vi "Analog IO.vi"(4 "R Audio In":i16, 5 "C O/P":i16[](array[numeric])=[0, 0], 6 "B O/P":u16[](array[numeric])=[0, 0, 0, 0], 7 "A O/P":u16[](array[numeric])=[0, 0, 0, 0]) -> (0 "R Audio Out":i16, 1 "C I/P":i16[](array[numeric]), 2 "B I/P":i16[](array[numeric]), 3 "A I/P":u16[](array[numeric]))   [LabVIEW 2015]
uses:
  <vilib>/rvi/eio/common/nirviEmuTemplateMethod_errors.vi
  <vilib>/eio/EIONode/EIONode.xnode
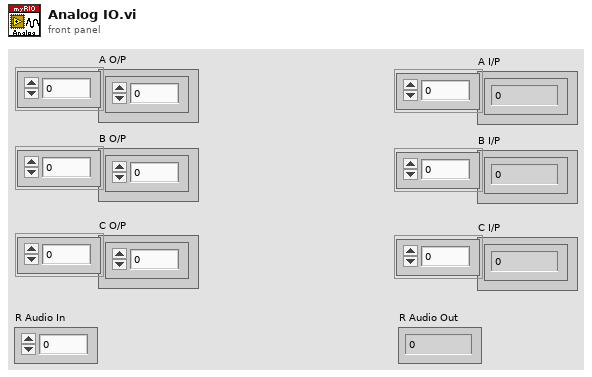
[diagram p1: front panel]
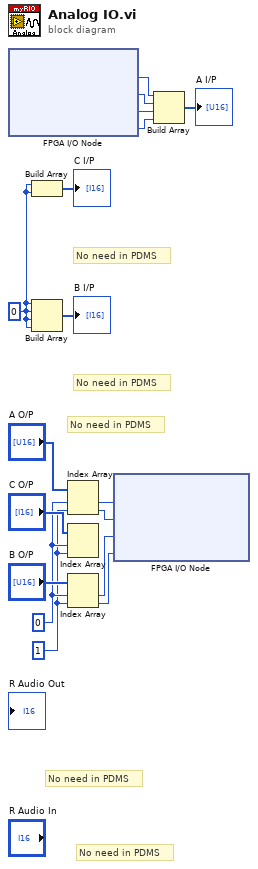
[diagram p0: block diagram]
diagram:
  w1 = i16 0
  w6 = i16 1
  w7 = i16 0
  # "No need in PDMS"
  # "No need in PDMS"
  # "No need in PDMS"
  # "No need in PDMS"
  # "No need in PDMS"
  n1 = xnode "FPGA I/O Node"() -> ("ConnectorA/AI0"=w17:u16, "ConnectorA/AI1"=w13:u16, "ConnectorA/AI2"=w12:u16, "ConnectorA/AI3"=w11:u16)  [unwired: 4 in, 4 out]
  n2 = Build Array(w1, w1) -> (→"C I/P":i16[])
  n3 = Build Array(w1, w1, w1, w1) -> (→"B I/P":i16[])
  n4 = Index Array(array="A O/P", index #1=w7, index #2=w6) -> (element #1=w5:u16, element #2=w4:u16)
  n5 = Index Array(array="C O/P", index #1=w7, index #2=w6) -> ()  [unwired: 2 out]
  n6 = Index Array(array="B O/P", index #1=w7, index #2=w6) -> (element #1=w3:u16, element #2=w2:u16)
  n7 = xnode "FPGA I/O Node"("ConnectorA/AO0"=w5, "ConnectorA/AO1"=w4, "ConnectorB/AO0"=w3, "ConnectorB/AO1"=w2) -> ()  [unwired: 4 in, 4 out]
  n8 = Build Array(w17, w13, w12, w11) -> (→"A I/P":u16[])
